vi "tc_color.vi"(10 "index (row)":i32, 11 "Color Box":u32(colorbox)=4250624) -> (3 "Thermocouples":T1(array[cluster]))   [LabVIEW 2017]
panel:
  in  "Numeric":dbl format="%#_13g"
  in  "initialized array":T1(array[cluster])
  in  "String":string
  in  "index (col)":i32
  out "Cluster":T2={"Numeric"=0.0, "Color Box"=12369084, "String"=""}
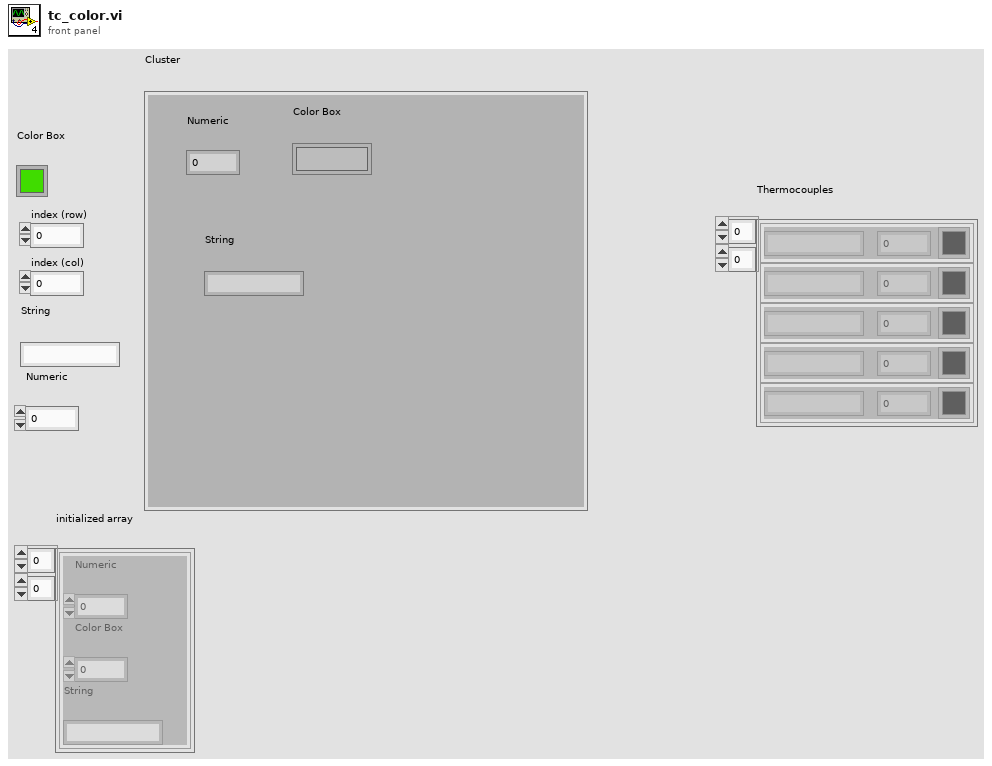
[diagram p1: front panel]
types:
  T1 = cluster{"Numeric":dbl, "Color Box":u32, "String":string}[][]
  T2 = cluster{"Numeric":dbl, "Color Box":u32, "String":string}
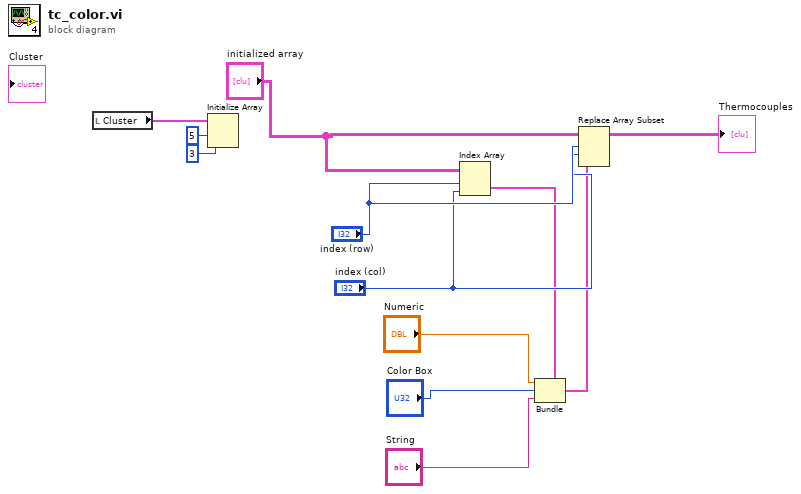
[diagram p0: block diagram]
diagram:
  n1 = local read "Cluster"() -> (w10:T2)
  n2 = Initialize Array(w10, 5 ("dimension size"), 3 ("dimension size")) -> ()  [unwired: 1 out]
  n3 = Index Array(array="initialized array", index (row)="index (row)", index (col)="index (col)") -> (element=w4:T2)
  n4 = Bundle(cluster=w4, "Numeric"="Numeric", "Color Box"="Color Box", "String"="String") -> (w5:T2)
  n5 = Replace Array Subset(array="initialized array", new element=w5, index (row)="index (row)", index (col)="index (col)") -> (→"Thermocouples":T1)
